vi "Parse.vi"(8 "error in (no error)":errorcluster, 10 "Transfer Group in":refnum<class "Transfer Group.lvclass">, 11 "Buffer Converter in":refnum<class "Buffer Converter.lvclass">) -> (0 "error out":errorcluster, 2 "Transfer Group out":refnum<class "Transfer Group.lvclass">, 3 "Buffer Converter out":refnum<class "Buffer Converter.lvclass">)   [LabVIEW 2017, in "DSF Core.lvlib" / "Buffer Converter.lvclass"]
uses:
  Buffer Converter.lvclass
  Transfer Group/Transfer Group.lvclass
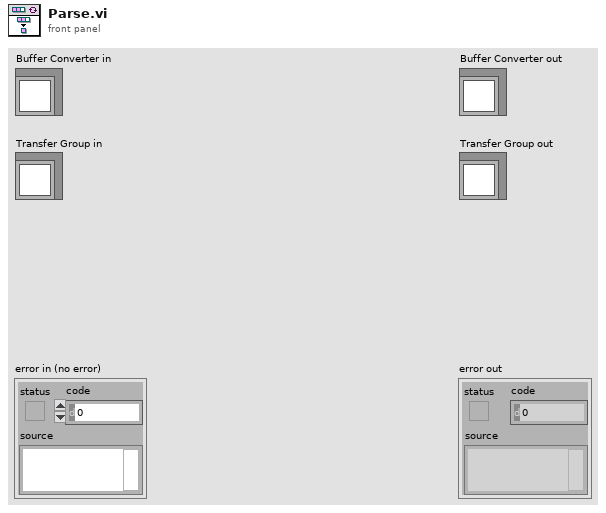
[diagram p1: front panel]
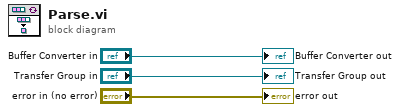
[diagram p0: block diagram]
diagram:
  "error out" <- "error in (no error)"
  "Buffer Converter out" <- "Buffer Converter in"
  "Transfer Group out" <- "Transfer Group in"
